vi "8.vi"() -> ()   [LabVIEW 2019]
panel:
  out "Waveform Graph":dynamicdata(graph)
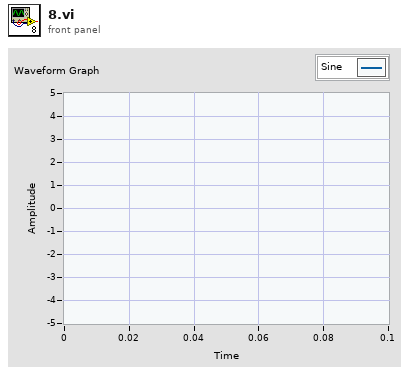
[diagram p1: front panel]
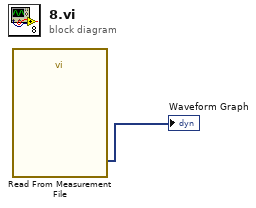
[diagram p0: block diagram]
diagram:
  n1 = call "Read From Measurement File"() -> ("Signals"=→"Waveform Graph":dynamicdata)  [unwired: 6 in, 5 out]
